vi "VCI_CAN_OBJ_N.vi"() -> ()   [LabVIEW 2017]
panel:
  out "VCI_CAN_OBJ_N":T1(array[cluster])
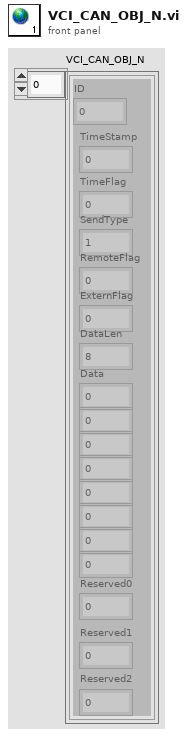
[diagram p1: front panel]
types:
  T1 = cluster{"ID":u32, "TimeStamp":u32, "TimeFlag":u8, "SendType":u8, "RemoteFlag":u8, "ExternFlag":u8, "DataLen":u8, "Data":u8, u8, u8, u8, u8, u8, u8, u8, "Reserved0":u8, "Reserved1":u8, "Reserved2":u8}[]
diagram:
